vi "CameraAbort.vi"(8 "error in":errorcluster, 11 "AndorSDK3 in":refnum<class "Andor3.lvclass">) -> (0 "error out":errorcluster, 3 "AndorSDK3 out":refnum<class "Andor3.lvclass">)   [LabVIEW 2010, in "Andor3.lvclass"]
uses:
  Andor3.lvclass
  Andor3.lvclass/Andor3.ctl
  <userlib>/atcoreA/atcoreA.lvlib
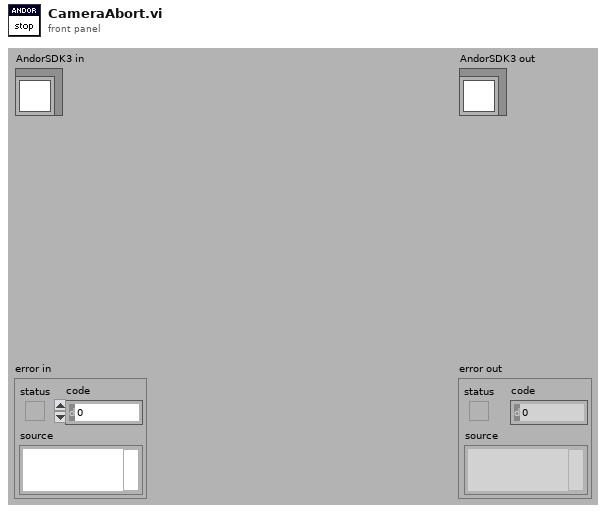
[diagram p1: front panel]
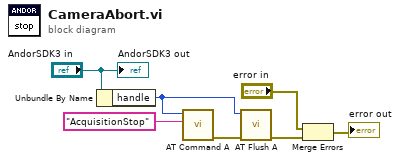
[diagram p0: block diagram]
diagram:
  n1 = Unbundle By Name("AndorSDK3 in") -> ("handle"=w4:i32)
  n2 = call <userlib>:"AT Command A.vi"("Feature"="AcquisitionStop", "Hndl"=w4) -> ("error out"=w5:errorcluster)  [unwired: 9 in]
  n3 = call <userlib>:"AT Flush A.vi"("error in (no error)"=w5, "Hndl"=w4) -> ("error out"=w3:errorcluster)  [unwired: 9 in]
  n4 = Merge Errors("error in", w3) -> (→"error out":errorcluster)
  "AndorSDK3 out" <- "AndorSDK3 in"
